vi "Day 6.vi"() -> ()   [LabVIEW 2019]
panel:
  out "Zones Under 10000":i32
  out "Largest Finite Area":i16
  out "Filtered Closest Point Indices":i32[][](array[numeric])
  out "Closest Point Indices":i32[][](array[numeric])
  out "Distances":i32[][][](array[numeric])
  out "Coordinates":i32[][](array[numeric])
  in  "Error In":errorcluster
  in  "Use Example Input":bool
  in  "Example Input":string="1, 1\n1, 6\n8, 3\n3, 4\n5, 5\n8, 9\n"
  in  "Relative Path to Input File":string="Day 6\\Day 6 Raw Input.txt"
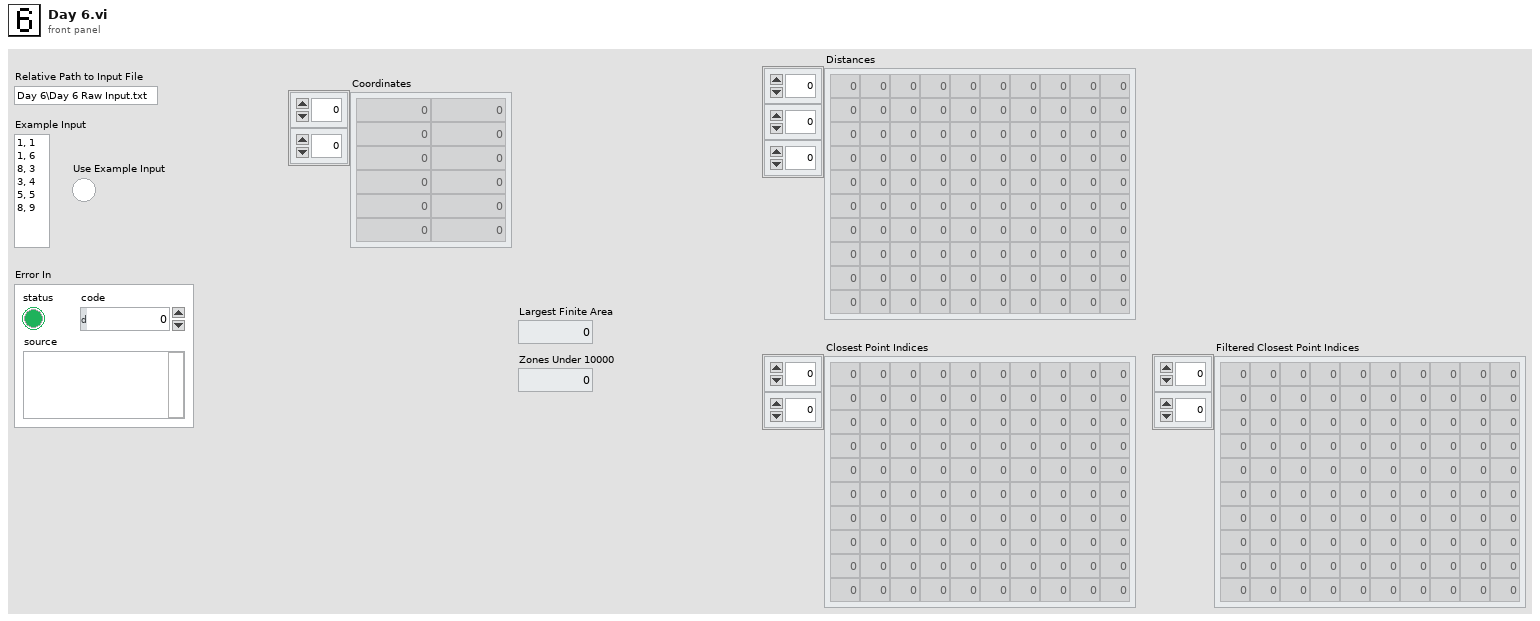
[diagram p1: front panel]
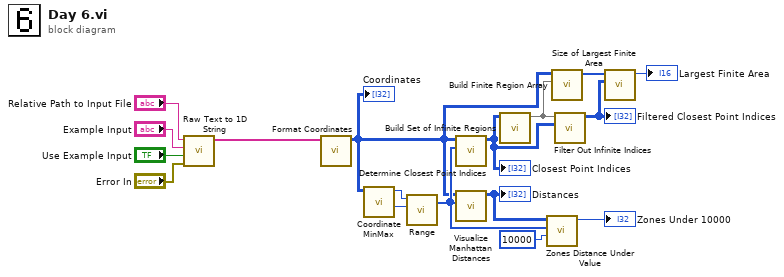
[diagram p0: block diagram]
diagram:
  n1 = call "Raw Text to 1D String.vi"("Error In"="Error In", "Use Example Input"="Use Example Input", "Example Input"="Example Input", "Relative Path to Input File"="Relative Path to Input File") -> ("1D String Array"=w13:string[])  [unwired: 6 in, 1 out]
  n2 = call "Format Coordinates.vi"("1D String Array"=w13) -> ("Coordinates"=w1:i32[][])  [unwired: 10 in]
  "Coordinates" <- w1
  n3 = call "Coordinate MinMax.vi"("Coordinates"=w1) -> ("Min Coordinate Value"=w3:i32, "Max Coordinate Value"=w12:i32)  [unwired: 9 in]
  n4 = call "Range.vi"("y"=w3, "x"=w12) -> ("Range"=w4:i32[])  [unwired: 5 in]
  n5 = call "Determine Closest Point Indices.vi"("Range"=w4, "Coordinates"=w1) -> ("Closest Point Indices"=w11:i32[][])  [unwired: 9 in]
  "Closest Point Indices" <- w11
  n6 = call "Visualize Manhattan Distances.vi"("Range"=w4, "Coordinates"=w1) -> ("Manhattan Distances"=w6:i32[][][])  [unwired: 9 in]
  "Distances" <- w6
  n7 = call "Build Set of Infinite Regions.vi"("Closest Point Indices"=w11) -> ("Infinite Regions"=w10:set{i32})  [unwired: 10 in]
  n8 = call "Zones Distance Under Value.vi"("Value"=10000, "Range"=w4, "Manhattan Distances"=w6) -> ("Numeric"=→"Zones Under 10000":i32)  [unwired: 8 in]
  n9 = call "Build Finite Region Array.vi"("Set"=w10, "Coordinates"=w1) -> ("Finite Regions"=w7:i32[])  [unwired: 9 in]
  n10 = call "Filter Out Infinite Indices.vi"("Closest Point Indices in"=w11, "Infinite Regions"=w10) -> ("Closest Point Indices out"=w9:i32[][])  [unwired: 9 in]
  "Filtered Closest Point Indices" <- w9
  n11 = call "Size of Largest Finite Area.vi"("Closest Point Indices in"=w9, "Finite Regions"=w7) -> ("Numeric"=→"Largest Finite Area":i16)  [unwired: 9 in]
